vi "Read Display Sec Listbox.vi"(8 "error in (no error)":errorcluster, 11 "GUI_Handler in":refnum<class "GUI_Handler.lvclass">) -> (0 "error out":errorcluster, 2 "Display Sec Listbox":refnum<vi>, 3 "GUI_Handler out":refnum<class "GUI_Handler.lvclass">)   [LabVIEW 2019, in "GUI_Handler.lvclass"]
uses:
  GUI_Handler.lvclass
  GUI_Handler.lvclass/GUI_Handler.ctl
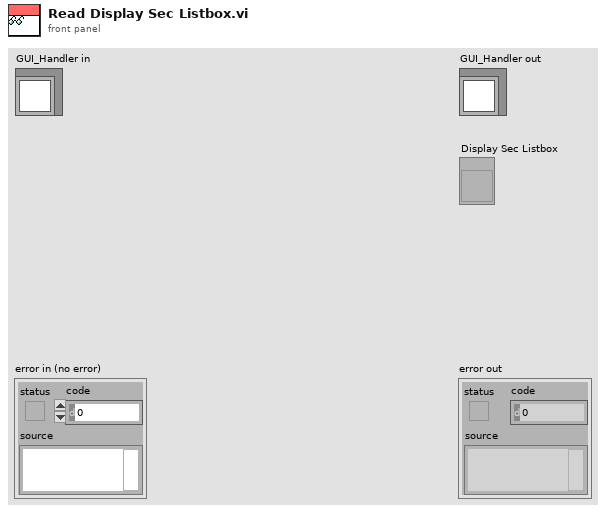
[diagram p1: front panel]
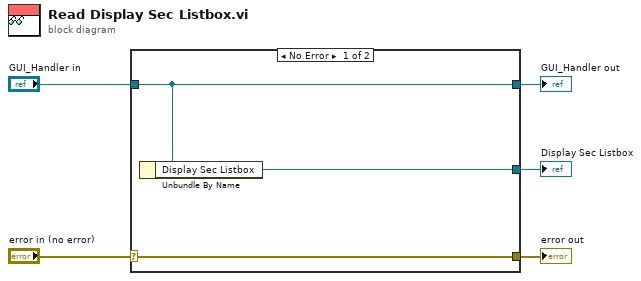
[diagram p0: block diagram]
diagram:
  n1 = case shown="No Error" "error in (no error)" {
    selector: "error in (no error)" -> [w8 w9]
    tunnel: [w8 w9] -> w4
    tunnel: [w7 w10] -> w2
    tunnel: "GUI_Handler in" -> [w7 w10]
    tunnel: [w6 _] -> w1
    frame No Error {
      n2 = Unbundle By Name(w7) -> ("Display Sec Listbox"=w6:refnum<vi>)
    }
    frame Error {
    }
  }
  "error out" <- w4
  "GUI_Handler out" <- w2
  "Display Sec Listbox" <- w1
